vi "Lab Final.vi"() -> ()   [LabVIEW 2015]
panel:
  in  "Cluster":T1
  out "String 10":string
  out "String 9":string
  out "String 8":string
  out "String 7":string
  out "Numeric 3":dbl
  out "Numeric 2":dbl
  out "Numeric":dbl
  out "Numeric":dbl
  out "String 4":string
  out "String 3":string
  out "String 2":string
  out "String":string
  out "L4":bool
  out "L3":bool
  out "L2":bool
  out "L1":bool
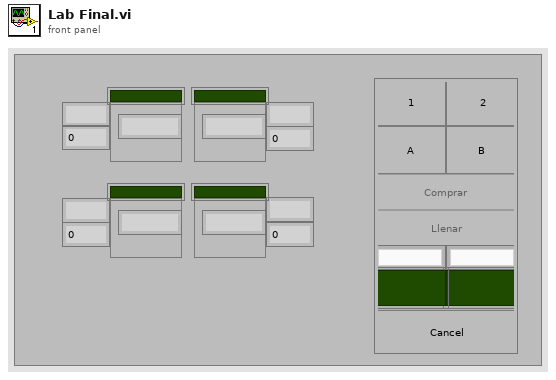
[diagram p1: front panel]
types:
  T1 = cluster{"1":bool, "2":bool, "B":bool, "A\n":bool, "Comprar":bool, "Llenar":bool, "Cancel Button":bool, "Boolean 5":bool, "Boolean 6":bool, "String 5":string, "String 6":string}
  T2 = enum8{"Enabled", "Disabled", "Disabled and Grayed Out"}
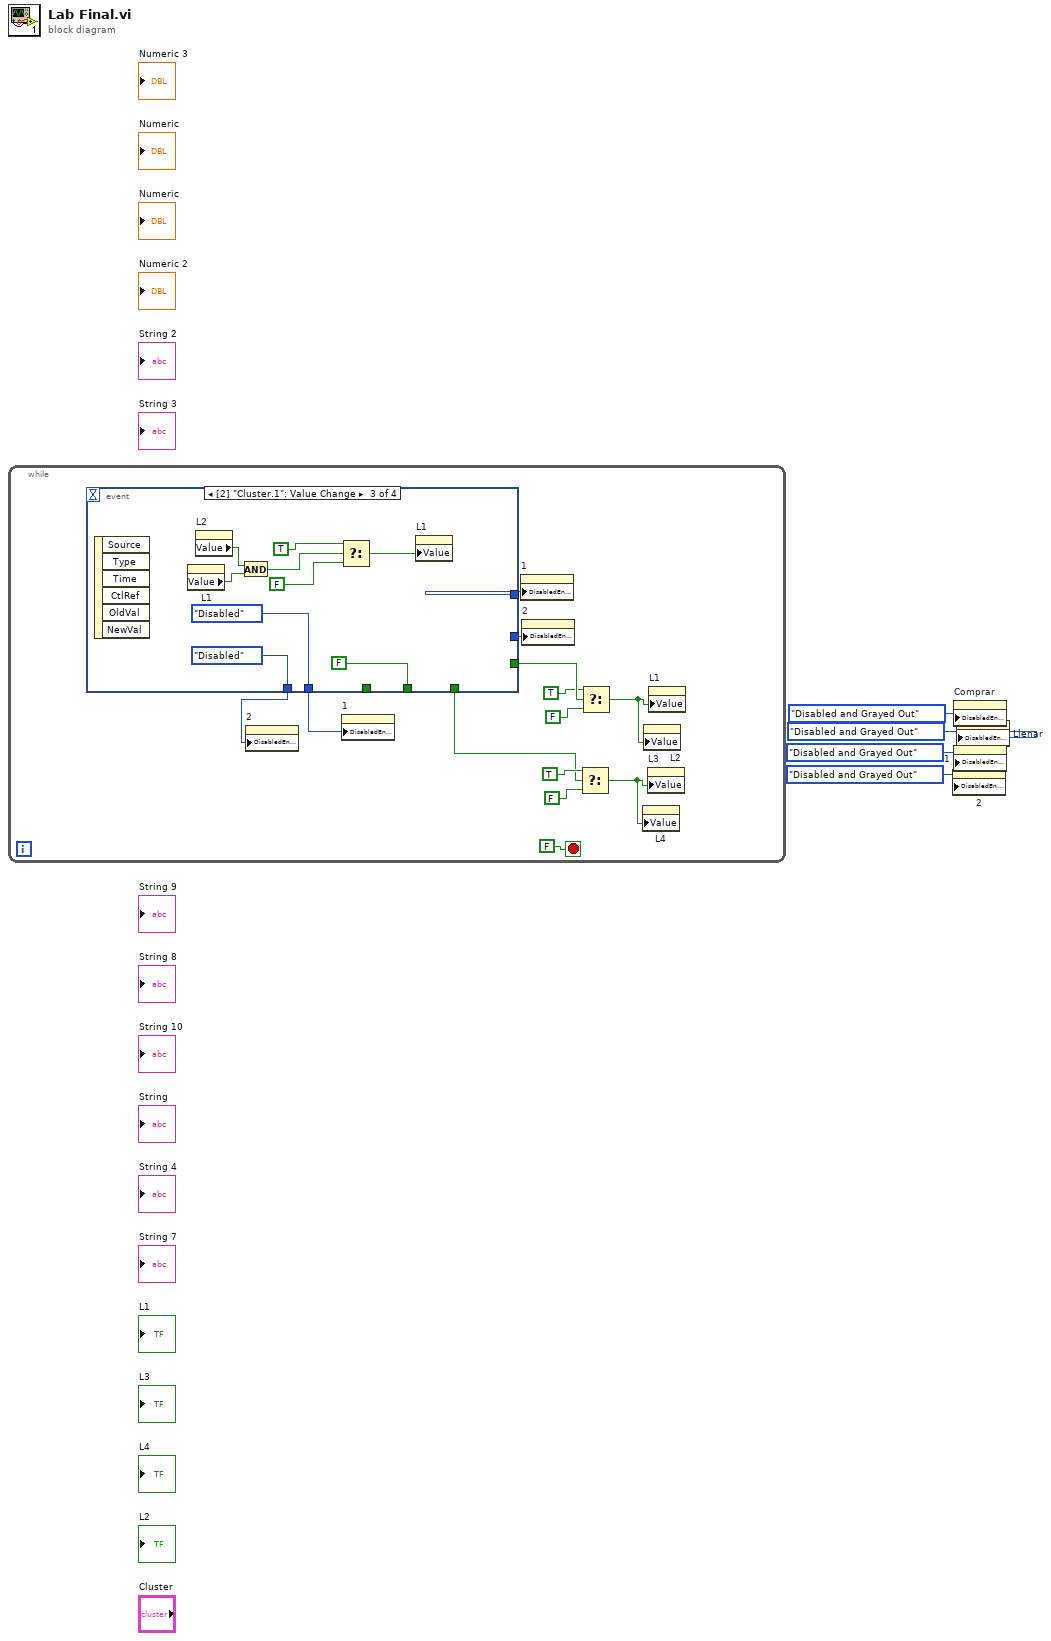
[diagram p0: block diagram]
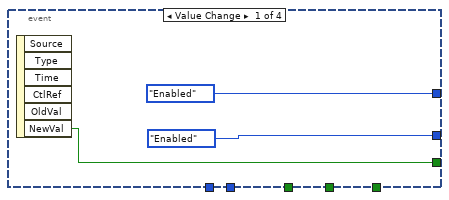
[diagram p2: hidden frame]
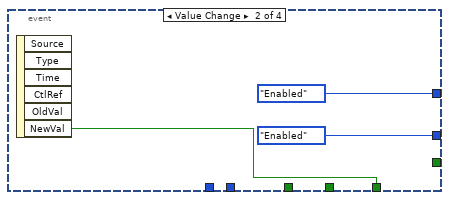
[diagram p3: hidden frame]
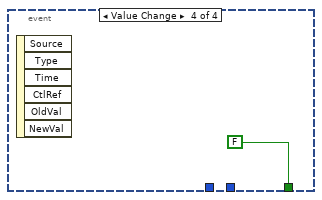
[diagram p4: hidden frame]
diagram:
  n1 = while {
    stop <- FALSE stop-if-true
    n2 = event shown="[2] \"Cluster.1\": Value Change" {
      selector: _ -> [_ _ _ _]
      dyn-events: _ -> [_ _ _ _]
      timeout: _ -> [_ _ _ _]
      tunnel: [T2."Enabled" ("Disabled") T2."Enabled" ("Disabled") _ _] -> w16
      tunnel: [T2."Enabled" ("Disabled") T2."Enabled" ("Disabled") _ _] -> w15
      tunnel: [_ _ T2."Disabled" ("Disabled") _] -> w14
      tunnel: [_ _ T2."Disabled" ("Disabled") _] -> w13
      tunnel: [_ _ FALSE _] -> _
      tunnel: [_ _ _ FALSE] -> _
      tunnel: [w18 _ _ _] -> w12
      tunnel: [_ w21 _ _] -> w5
      event "Cluster.A": Value Change {
        n3 = event-data() -> ("NewVal"=w18:bool)  [unwired: 1 in, 5 out]
      }
      event "Cluster.B": Value Change {
        n4 = event-data() -> ("NewVal"=w21:bool)  [unwired: 1 in, 5 out]
      }
      event "Cluster.1": Value Change {
        n5 = event-data() -> ()  [unwired: 1 in, 6 out]
        n6 = property on="L1" class="Bool (strict)"() -> ("Value"=w27:bool)  [unwired: 2 in, 2 out]
        n7 = property on="L2" class="Bool (strict)"() -> ("Value"=w26:bool)  [unwired: 2 in, 2 out]
        n8 = And(x=w26, y=w27) -> (x .and. y?=w25:bool)
        n9 = Select(t=TRUE, s=w25, f=FALSE) -> (s? t:f=w24:bool)
        n10 = property on="L1" class="Bool (strict)"("Value"=w24) -> ()  [unwired: 2 in, 2 out]
      }
      event "Cluster.2": Value Change {
        n11 = event-data() -> ()  [unwired: 1 in, 6 out]
      }
    }
    n12 = property on="2" class="Bool"("DisabledEnum"=w13) -> ()  [unwired: 2 in, 2 out]
    n13 = property on="1" class="Bool"("DisabledEnum"=w14) -> ()  [unwired: 2 in, 2 out]
    n14 = property on="1" class="Bool"("DisabledEnum"=w16) -> ()  [unwired: 2 in, 2 out]
    n15 = property on="2" class="Bool"("DisabledEnum"=w15) -> ()  [unwired: 2 in, 2 out]
    n16 = Select(t=TRUE, s=w5, f=FALSE) -> (s? t:f=w6:bool)
    n17 = Select(t=TRUE, s=w12, f=FALSE) -> (s? t:f=w9:bool)
    n18 = property on="L4" class="Bool (strict)"("Value"=w6) -> ()  [unwired: 2 in, 2 out]
    n19 = property on="L2" class="Bool (strict)"("Value"=w9) -> ()  [unwired: 2 in, 2 out]
    n20 = property on="L3" class="Bool (strict)"("Value"=w6) -> ()  [unwired: 2 in, 2 out]
    n21 = property on="L1" class="Bool (strict)"("Value"=w9) -> ()  [unwired: 2 in, 2 out]
  }
  n22 = property on="2" class="Bool"("DisabledEnum"=T2."Disabled and Grayed Out" ("Disabled")) -> ()  [unwired: 2 in, 2 out]
  n23 = property on="Comprar" class="Bool (strict)"("DisabledEnum"=T2."Disabled and Grayed Out" ("Disabled")) -> ()  [unwired: 2 in, 2 out]
  n24 = property on="1" class="Bool"("DisabledEnum"=T2."Disabled and Grayed Out" ("Disabled")) -> ()  [unwired: 2 in, 2 out]
  n25 = property on="Llenar" class="Bool"("DisabledEnum"=T2."Disabled and Grayed Out" ("Disabled")) -> ()  [unwired: 2 in, 2 out]
